vi "Error Handler.vi"(8 "error in (no error)":errorcluster, 10 "clear inline error? (F)":bool, 11 "Framework in":refnum<class "Framework.lvclass">) -> (0 "error out":errorcluster, 3 "Framework out":refnum<class "Framework.lvclass">)   [LabVIEW 2021, in "DSF Core.lvlib" / "Framework.lvclass"]
uses:
  Framework.lvclass
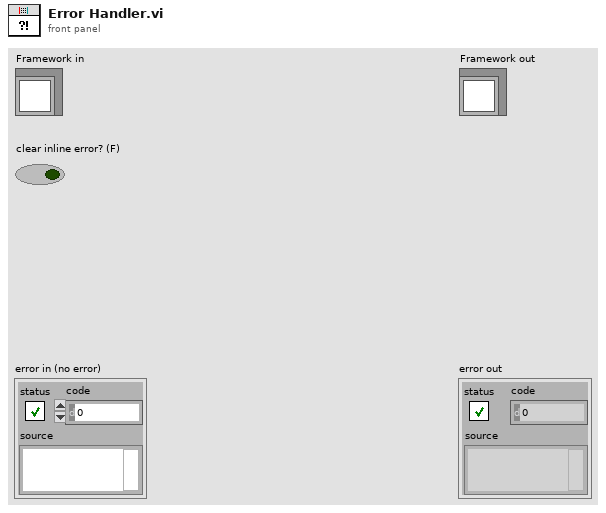
[diagram p1: front panel]
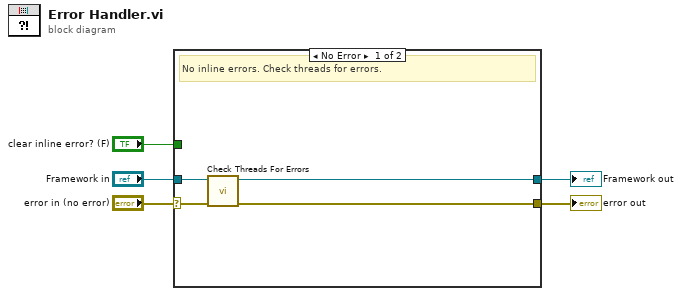
[diagram p0: block diagram]
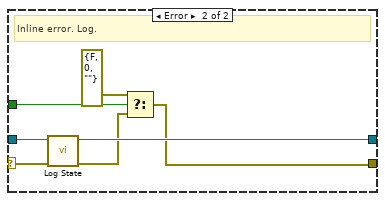
[diagram p2: hidden frame]
diagram:
  n1 = case shown="No Error" "error in (no error)" {
    selector: "error in (no error)" -> [w9 w15]
    tunnel: "Framework in" -> [w8 w14]
    tunnel: [w6 w13] -> w4
    tunnel: [w7 w10] -> w3
    tunnel: "clear inline error? (F)" -> [_ w16]
    frame No Error {
      # "No inline errors. Check threads for errors."
      n2 = call "Check Threads For Errors.vi"("error in (no error)"=w9, "Framework in"=w8) -> ("error out"=w7:errorcluster, "Framework out"=w6:refnum<class "Framework.lvclass">)  [unwired: 6 in, 2 out]
    }
    frame Error {
      # "Inline error. Log."
      n3 = call "Log State.vi"("error in (no error)"=w15, "Framework in"=w14) -> ("error out"=w11:errorcluster, "Framework out"=w13:refnum<class "Framework.lvclass">)  [unwired: 8 in]
      n4 = Select(t=errorcluster {"status"=FALSE, "code"=0, "source"=""}, s=w16, f=w11) -> (s? t:f=w10:errorcluster)
    }
  }
  "error out" <- w3
  "Framework out" <- w4
